vi "Status Monitor (Single Unit).vi"(9 "Update Status Event":refnum<user-event>, 10 "Device Index":i32, 11 "configuration file path":path) -> ()   [LabVIEW 2017, in "Status Monitor Library.lvlib"]
doc: "Connects to the status port and frequently reads the buffer. \n\nAttempts to decode that data in a status message. If the decoding is sucessful, a user event is triggered and that status message is made available through the event."
uses:
  Status Monitor Library.lvlib
  Combined Status and Transient/SubVIs/Device Status and Index--Cluster.ctl
  Communications/Typedefs/DTACQ Module Carrier Status.ctl
  Communications/Typedefs/DTACQ Status--Enum.ctl
  Communications/Communications Library.lvlib
panel:
  in  "Stop":bool
  out "Demuxing":bool
  out "Total Samples":i32
  out "Post-Buffered Samples":i32
  out "Pre-Buffered Samples":i32
  out "Device State":T1(ring)
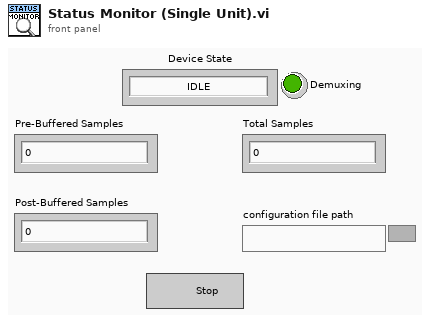
[diagram p1: front panel]
types:
  T1 = enum16{"IDLE", "ARM", "RUN_PRE-TRIGGER", "RUN_POST-TRIGGER", "POST_PROCESS", "CLEANUP"}
  T2 = typedef "Communications Library.lvlib/DTACQ Module Carrier Configuration--Cluster.ctl" = cluster{"Name":string, "IP":string, "Control Port":i32, "Timeout (ms)":i32, "Continuous Capture Port (Multiplexed)":i32, "Start HIL Shot Port":i32, "AWG Upload Port (Multiplexed)":i32, "Download Captured Data Port (Multiplexed)":i32, "Module Slots":i32, "Module Configurations":T3[]}
  T3 = typedef "Communications Library.lvlib/DTACQ Module Configuration--Cluster.ctl" = cluster{"Name":string, "Position":string, "Module Type":T4, "Control Port":i32, "Timeout (ms)":i32, "Channels":i32}
  T4 = typedef "Communications Library.lvlib/DTACQ Device Type--Enum.ctl" = enum16{"Carrier", "Analog In Module", "Analog Out Module", "Generic Module"}
  T5 = typedef "Communications Library.lvlib/DTACQ Connection Data--Cluster.ctl" = cluster{"Description":string, "Address":string, "Port":u16, "timeout (ms)":i32, "Termination Character":string, "TCP Connection Reference":refnum<k5>, "Open Connection":bool}
  T6 = typedef "Device Status and Index--Cluster.ctl" = cluster{"Device Index":i32, "Module Carrier Status":T7}
  T7 = typedef "Communications Library.lvlib/DTACQ Module Carrier Status.ctl" = cluster{"DTACQ State":T8, "Pre-Trigger Samples":i32, "Post-Trigger Samples":i32, "Total Samples":i32, "Post Processing":bool}
  T8 = typedef "Communications Library.lvlib/DTACQ Status--Enum.ctl" = enum16{"IDLE", "ARM", "RUN_PRE-TRIGGER", "RUN_POST-TRIGGER", "POST_PROCESS", "CLEANUP"}
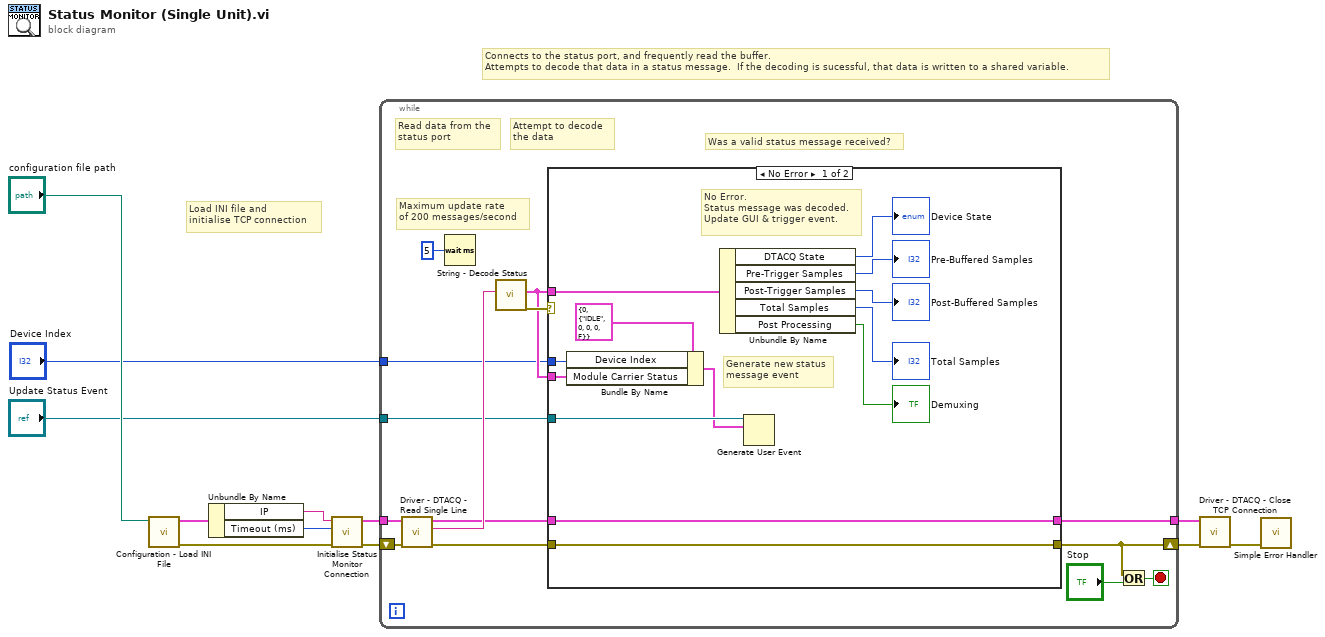
[diagram p0: block diagram]
diagram:
  # "Connects to the status port, and frequently read the buffer.  \nAttempts to decode that data in a status message.  If the decoding is sucessful, that data is written to a shared variable."
  # "Load INI file and\ninitialise TCP connection"
  n1 = call "Configuration - Load INI File.vi"("configuration file path"="configuration file path") -> ("error out"=w7:errorcluster, "Carrier Configuration Out"=w9:T2)  [unwired: 9 in]
  n2 = Unbundle By Name(w9) -> ("IP"=w8:string, "Timeout (ms)"=w6:i32)
  n3 = call "Initialise Status Monitor Connection.vi"("error in"=w7, "timeout (ms)"=w6, "Address"=w8) -> ("error out"=w4:errorcluster, "Status Connection Out"=w12:T5)  [unwired: 7 in]
  n4 = while {
    tunnel: w12 -> [w26]
    shift-right: [w17] -> w11
    shift-left: w4 -> [w24]
    tunnel: [w15] -> w10
    tunnel: "Update Status Event" -> [w14]
    tunnel: "Device Index" -> [w13]
    stop <- w22 stop-if-true
    # "Was a valid status message received?"
    # "Attempt to decode\nthe data"
    # "Read data from the\nstatus port"
    # "Maximum update rate\nof 200 messages/second"
    n5 = call "Driver - DTACQ - Read Single Line.vi"("error in"=w24, "DTACQ Connection Data In"=w26) -> ("error out"=w18:errorcluster, "Read String"=w25:string, "DTACQ Connection Data Out"=w16:T5)  [unwired: 6 in, 1 out]
    n6 = Wait (ms)(milliseconds to wait=u32 5) -> ()  [unwired: 1 out]
    n7 = call "String - Decode Status.vi"("Status Response String"=w25) -> ("error out"=w23:errorcluster, "Module Carrier Status"=w19:T7)  [unwired: 9 in]
    n8 = case shown="No Error" w23 {
      tunnel: w19 -> [w32 _]
      tunnel: w19 -> [w27 _]
      tunnel: w18 -> [w31 w41]
      tunnel: [w31 w41] -> w17
      tunnel: w16 -> [w34 w40]
      tunnel: [w34 w40] -> w15
      tunnel: w14 -> [w33 _]
      tunnel: w13 -> [w29 _]
      frame No Error {
        # "Generate new status\nmessage event"
        # "No Error.\nStatus message was decoded.\nUpdate GUI & trigger event."
        n9 = Bundle By Name(cluster=T6 {"Device Index"=0, "Module Carrier Status"={"DTACQ State"=enum."IDLE", "Pre-Trigger Samples"=0, "Post-Trigger Samples"=0, "Total Samples"=0, "Post Processing"=FALSE}} ("Device Status and Index"), "Device Index"=w29, "Module Carrier Status"=w27) -> (w28:T6)
        n10 = Unbundle By Name(w32) -> ("DTACQ State"=→"Device State":T8, "Pre-Trigger Samples"=→"Pre-Buffered Samples":i32, "Post-Trigger Samples"=→"Post-Buffered Samples":i32, "Total Samples"=→"Total Samples":i32, "Post Processing"=→"Demuxing":bool)
        n11 = Generate User Event(user event=w33, event data cluster=w28) -> ()  [unwired: 2 in, 2 out]
      }
      frame Error {
        # "Error decoding message.\nNot a valid status message,\nso leave the GUI as-is."
      }
    }
    n12 = Or(x=w17, y="Stop") -> (x .or. y?=w22:bool)
  }
  n13 = call "Driver - DTACQ - Close TCP Connection.vi"("error in"=w11, "DTACQ Connection Data In"=w10) -> ("error out"=w1:errorcluster)  [unwired: 8 in, 1 out]
  n14 = call <vilib>:"Simple Error Handler.vi"("error in (no error)"=w1) -> ()  [unwired: 4 in, 5 out]
